vi "AVG Vrms.vi"(9 "Line 3":waveform(dbl), 10 "Line 2":waveform(dbl), 11 "Line 1":waveform(dbl)) -> (3 "AVG RMS":dbl)   [LabVIEW 2019]
uses:
  <vilib>/measure/madcrms.llb/Basic Averaged DC-RMS for 1 Chan.vi
  <vilib>/measure/NI_MAPro.lvlib
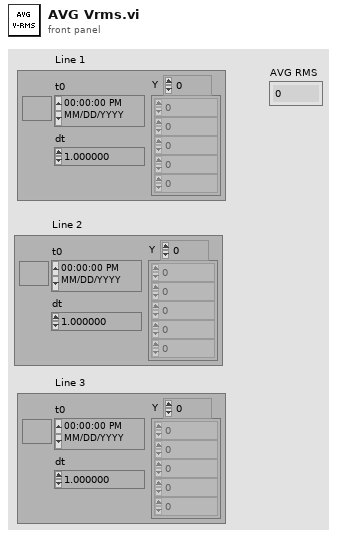
[diagram p1: front panel]
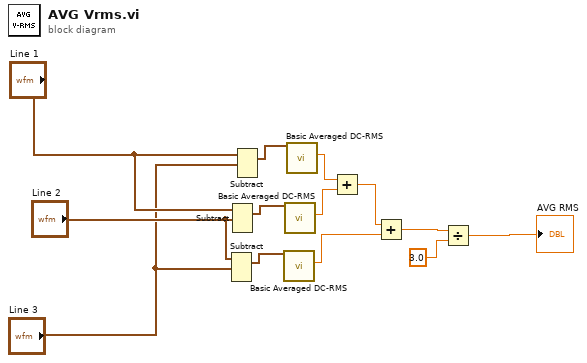
[diagram p0: block diagram]
diagram:
  n1 = Subtract(1:"Line 3", 2:"Line 2") -> (0:w1:waveform(dbl))  [unwired: 1 in, 1 out]
  n2 = Subtract(1:"Line 2", 2:"Line 1") -> (0:w6:waveform(dbl))  [unwired: 1 in, 1 out]
  n3 = Subtract(1:"Line 3", 2:"Line 1") -> (0:w7:waveform(dbl))  [unwired: 1 in, 1 out]
  n4 = call-poly <vilib>:"Basic Averaged DC-RMS.vi"("signal in"=w1) -> ("RMS value"=w10:dbl)  [unwired: 7 in, 3 out]
  n5 = call-poly <vilib>:"Basic Averaged DC-RMS.vi"("signal in"=w6) -> ("RMS value"=w12:dbl)  [unwired: 7 in, 3 out]
  n6 = call-poly <vilib>:"Basic Averaged DC-RMS.vi"("signal in"=w7) -> ("RMS value"=w13:dbl)  [unwired: 7 in, 3 out]
  n7 = Add(x=w13, y=w12) -> (x+y=w11:dbl)
  n8 = Add(x=w11, y=w10) -> (x+y=w9:dbl)
  n9 = Divide(x=w9, y=3.0) -> (x/y=→"AVG RMS":dbl)
